vi "Calc Lift Speeds.vi"(9 "Joystick Axes":dbl[](array[numeric]), 10 "Lower Limit Switch":bool, 11 "Upper Limit Switch":bool) -> (3 "Lift Speed":dbl)   [LabVIEW 2018]
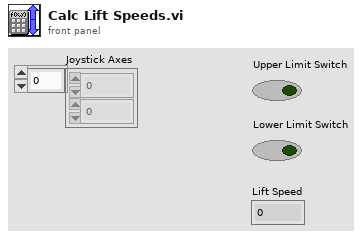
[diagram p1: front panel]
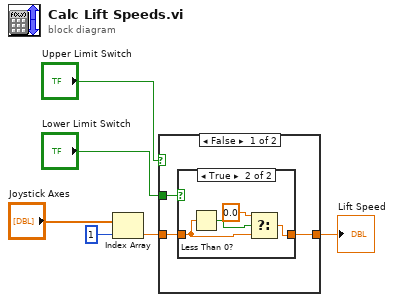
[diagram p0: block diagram]
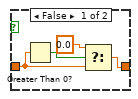
[diagram p4: hidden frame]
diagram:
  n1 = Index Array(array="Joystick Axes", index=1) -> (element=w3:dbl)
  n2 = case shown="False" "Upper Limit Switch" {
    tunnel: w3 -> [w9 w17]
    tunnel: [w8 w16] -> w2
    tunnel: "Lower Limit Switch" -> [w7 w15]
    frame False {
      n3 = case shown="True" w7 {
        tunnel: w9 -> [w10 w12]
        tunnel: [w10 w11] -> w8
        frame False {
        }
        frame True {
          n4 = Less Than 0?(x=w12) -> (x < 0?=w14:bool)
          n5 = Select(t=0.0, s=w14, f=w12) -> (s? t:f=w11:dbl)
        }
      }
    }
    frame True {
      n6 = case shown="True" w15 {
        tunnel: w17 -> [w19 w22]
        tunnel: [w18 w22] -> w16
        frame False {
          n7 = Greater Than 0?(x=w19) -> (x > 0?=w21:bool)
          n8 = Select(t=0.0, s=w21, f=w19) -> (s? t:f=w18:dbl)
        }
        frame True {
        }
      }
    }
  }
  "Lift Speed" <- w2
